vi "test_read-nmea-data2.vi"() -> ()   [LabVIEW 2019] (continued)
$GAGSV,2,1,08,02,08,297,,04,66,118,20,09,32,193,,11,71,358,,2*7E\n\t\n15:11:17.65\tF9P\t$GAGSV,2,2,08,12,40,102,24,19,26,045,24,25,09,249,,36,26,308,,2*7C\n\t\n15:11:17.67\tF9P\t$GBGSV,1,1,03,11,50,131,24,14,87,138,31,33,60,219,26,1*4F\n\t\n15:11:17.69\tF9P\t$GBGSV,1,1,03,11,50,131,31,14,87,138,23,33,60,219,,3*4E\n\t\n15:11:17.71\tF9P\t$GNGLL,3723.53985,N,12656.90241,E,061119.00,A,A*76\n\t\n15:11:17.73\tF9P\t\t\n15:11:17.75\tF9P\t\t\n15:11:17.77\tF9P\t\t\n15:11:17.79\tF9P\t\t\n15:11:17.81\tF9P\t\t\n15:11:17.83\tF9P\t\t\n15:11:17.85\tF9P\t\t\n15:11:17.87\tF9P\t\t\n15:11:17.89\tF9P\t\t\n15:11:17.91\tF9P\t\t\n15:11:17.93\tF9P\t\t\n15:11:17.95\tF9P\t\t\n15:11:17.97\tF9P\t\t\n15:11:17.99\tF9P\t\t\n15:11:18.01\tF9P\t\t\n15:11:18.03\tF9P\t\t\n15:11:18.05\tF9P\t\t\n15:11:18.07\tF9P\t\t\n15:11:18.09\tF9P\t\t\n15:11:18.11\tF9P\t\t\n15:11:18.13\tF9P\t\t\n15:11:18.15\tF9P\t\t\n15:11:18.17\tF9P\t\t\n15:11:18.19\tF9P\t\t\n15:11:18.21\tF9P\t\t\n15:11:18.23\tF9P\t\t\n15:11:18.25\tF9P\t$GNRMC,061120.00,A,3723.53889,N,12656.90285,E,2.155,137.19,250720,,,A,V*08\n\t\n15:11:18.27\tF9P\t$GNVTG,137.19,T,,M,2.155,N,3.990,K,A*2E\n\t\n15:11:18.29\tF9P\t$GNGGA,061120.00,3723.53889,N,12656.90285,E,1,12,0.68,42.0,M,18.5,M,,*7B\n\t\n15:11:18.31\tF9P\t$GNGSA,A,3,12,06,19,05,17,09,04,02,,,,,1.27,0.68,1.08,1*03\n\t\n15:11:18.33\tF9P\t$GNGSA,A,3,85,71,84,,,,,,,,,,1.27,0.68,1.08,2*06\n\t\n15:11:18.35\tF9P\t$GNGSA,A,3,36,19,11,04,09,12,,,,,,,1.27,0.68,1.08,3*03\n\t\n15:11:18.37\tF9P\t$GNGSA,A,3,14,11,33,,,,,,,,,,1.27,0.68,1.08,4*02\n\t\n15:11:18.39\tF9P\t$GPGSV,3,1,09,02,54,318,32,04,18,044,24,05,37,247,29,06,64,047,35,1*66\n\t\n15:11:18.41\tF9P\t$GPGSV,3,2,09,09,45,074,31,12,24,277,21,17,33,153,38,19,53,157,29,1*6D\n\t\n15:11:18.43\tF9P\t$GPGSV,3,3,09,25,12,307,16,1*5A\n\t\n15:11:18.45\tF9P\t$GPGSV,3,1,09,02,54,318,,04,18,044,21,05,37,247,,06,64,047,,6*68\n\t\n15:11:18.47\tF9P\t$GPGSV,3,2,09,09,45,074,23,12,24,277,,17,33,153,21,19,53,157,,6*69\n\t\n15:11:18.49\tF9P\t$GPGSV,3,3,09,25,12,307,,6*5A\n\t\n15:11:18.51\tF9P\t$GLGSV,2,1,08,69,12,031,,70,72,041,,71,51,205,20,72,03,209,,1*70\n\t\n15:11:18.53\tF9P\t$GLGSV,2,2,08,77,01,326,,84,20,122,10,85,70,065,23,86,36,330,,1*7B\n\t\n15:11:18.55\tF9P\t$GLGSV,2,1,08,69,12,031,,70,72,041,,71,51,205,15,72,03,209,,3*74\n\t\n15:11:18.57\tF9P\t$GLGSV,2,2,08,77,01,326,,84,20,122,18,85,70,065,20,86,36,330,,3*72\n\t\n15:11:18.59\tF9P\t$GAGSV,2,1,08,02,08,297,06,04,66,118,31,09,32,193,31,11,71,358,23,7*7E\n\t\n15:11:18.61\tF9P\t$GAGSV,2,2,08,12,40,102,22,19,26,045,22,25,09,249,,36,26,308,38,7*72\n\t\n15:11:18.63\tF9P\t$GAGSV,2,1,08,02,08,297,,04,66,118,20,09,32,193,,11,71,358,,2*7E\n\t\n15:11:18.65\tF9P\t$GAGSV,2,2,08,12,40,102,23,19,26,045,22,25,09,249,,36,26,308,,2*7D\n\t\n15:11:18.67\tF9P\t$GBGSV,1,1,03,11,50,132,24,14,87,138,26,33,60,219,25,1*49\n\t\n15:11:18.69\tF9P\t$GBGSV,1,1,03,11,50,132,24,14,87,138,22,33,60,219,,3*48\n\t\n15:11:18.71\tF9P\t$GNGLL,3723.53889,N,12656.90285,E,061120.00,A,A*79\n\t\n15:11:18.73\tF9P\t\t\n15:11:18.75\tF9P\t\t\n15:11:18.77\tF9P\t\t\n15:11:18.79\tF9P\t\t\n15:11:18.81\tF9P\t\t\n15:11:18.83\tF9P\t\t\n15:11:18.85\tF9P\t\t\n15:11:18.87\tF9P\t\t\n15:11:18.89\tF9P\t\t\n15:11:18.91\tF9P\t\t\n15:11:18.93\tF9P\t\t\n15:11:18.95\tF9P\t\t\n15:11:18.97\tF9P\t\t\n15:11:18.99\tF9P\t\t\n15:11:19.01\tF9P\t\t\n15:11:19.03\tF9P\t\t\n15:11:19.05\tF9P\t\t\n15:11:19.07\tF9P\t\t\n15:11:19.09\tF9P\t\t\n15:11:19.11\tF9P\t\t\n15:11:19.13\tF9P\t\t\n15:11:19.15\tF9P\t\t\n15:11:19.17\tF9P\t\t\n15:11:19.19\tF9P\t\t\n15:11:19.21\tF9P\t\t\n15:11:19.23\tF9P\t\t\n15:11:19.25\tF9P\t$GNRMC,061121.00,A,3723.53803,N,12656.90342,E,2.573,139.60,250720,,,A,V*01\n\t\n15:11:19.27\tF9P\t$GNVTG,139.60,T,,M,2.573,N,4.764,K,A*2C\n\t\n15:11:19.29\tF9P\t$GNGGA,061121.00,3723.53803,N,12656.90342,E,1,12,0.68,40.8,M,18.5,M,,*78\n\t\n15:11:19.31\tF9P\t$GNGSA,A,3,12,06,19,05,17,09,04,02,,,,,1.27,0.68,1.08,1*03\n\t\n15:11:19.33\tF9P\t$GNGSA,A,3,85,71,84,,,,,,,,,,1.27,0.68,1.08,2*06\n\t\n15:11:19.35\tF9P\t$GNGSA,A,3,36,19,11,04,09,12,,,,,,,1.27,0.68,1.08,3*03\n\t\n15:11:19.37\tF9P\t$GNGSA,A,3,14,11,33,,,,,,,,,,1.27,0.68,1.08,4*02\n\t\n15:11:19.39\tF9P\t$GPGSV,3,1,09,02,54,318,32,04,18,044,25,05,37,247,28,06,64,047,30,1*63\n\t\n15:11:19.41\tF9P\t$GPGSV,3,2,09,09,45,074,27,12,24,277,22,17,33,153,36,19,53,157,33,1*6C\n\t\n15:11:19.43\tF9P\t$GPGSV,3,3,09,25,12,307,16,1*5A\n\t\n15:11:19.45\tF9P\t$GPGSV,3,1,09,02,54,318,,04,18,044,21,05,37,247,,06,64,047,19,6*60\n\t\n15:11:19.47\tF9P\t$GPGSV,3,2,09,09,45,074,19,12,24,277,,17,33,153,22,19,53,157,,6*63\n\t\n15:11:19.49\tF9P\t$GPGSV,3,3,09,25,12,307,,6*5A\n\t\n15:11:19.51\tF9P\t$GLGSV,2,1,08,69,12,031,,70,72,041,,71,51,205,19,72,03,209,,1*7A\n\t\n15:11:19.53\tF9P\t$GLGSV,2,2,08,77,01,326,,84,20,122,10,85,70,065,23,86,36,330,,1*7B\n\t\n15:11:19.55\tF9P\t$GLGSV,2,1,08,69,12,031,,70,72,041,,71,51,205,16,72,03,209,,3*77\n\t\n15:11:19.57\tF9P\t$GLGSV,2,2,08,77,01,326,,84,20,122,18,85,70,065,19,86,36,330,,3*78\n\t\n15:11:19.59\tF9P\t$GAGSV,2,1,08,02,08,297,10,04,66,118,30,09,32,193,30,11,71,358,28,7*72\n\t\n15:11:19.61\tF9P\t$GAGSV,2,2,08,12,40,102,21,19,26,045,22,25,09,249,,36,26,308,23,7*7B\n\t\n15:11:19.63\tF9P\t$GAGSV,2,1,08,02,08,297,,04,66,118,20,09,32,193,,11,71,358,,2*7E\n\t\n15:11:19.65\tF9P\t$GAGSV,2,2,08,12,40,102,23,19,26,045,18,25,09,249,,36,26,308,,2*74\n\t\n15:11:19.67\tF9P\t$GBGSV,1,1,03,11,50,132,24,14,87,127,23,33,60,219,23,1*44\n\t\n15:11:19.69\tF9P\t$GBGSV,1,1,03,11,50,132,25,14,87,127,22,33,60,219,,3*47\n\t\n15:11:19.71\tF9P\t$GNGLL,3723.53803,N,12656.90342,E,061121.00,A,A*70\n\t\n15:11:19.73\tF9P\t\t\n15:11:19.75\tF9P\t\t\n15:11:19.77\tF9P\t\t\n15:11:19.79\tF9P\t\t\n15:11:19.81\tF9P\t\t\n15:11:19.83\tF9P\t\t\n15:11:19.85\tF9P\t\t\n15:11:19.87\tF9P\t\t\n15:11:19.89\tF9P\t\t\n15:11:19.91\tF9P\t\t\n15:11:19.93\tF9P\t\t\n15:11:19.95\tF9P\t\t\n15:11:19.97\tF9P\t\t\n15:11:19.99\tF9P\t\t\n15:11:20.01\tF9P\t\t\n15:11:20.03\tF9P\t\t\n15:11:20.05\tF9P\t\t\n15:11:20.07\tF9P\t\t\n15:11:20.09\tF9P\t\t\n15:11:20.11\tF9P\t\t\n15:11:20.13\tF9P\t\t\n15:11:20.15\tF9P\t\t\n15:11:20.17\tF9P\t\t\n15:11:20.19\tF9P\t\t\n15:11:20.21\tF9P\t\t\n15:11:20.23\tF9P\t\t\n15:11:20.25\tF9P\t$GNRMC,061122.00,A,3723.53728,N,12656.90355,E,1.979,141.75,250720,,,A,V*0C\n\t\n15:11:20.27\tF9P\t$GNVTG,141.75,T,,M,1.979,N,3.666,K,A*26\n\t\n15:11:20.29\tF9P\t$GNGGA,061122.00,3723.53728,N,12656.90355,E,1,12,0.67,41.8,M,18.5,M,,*75\n\t\n15:11:20.31\tF9P\t$GNGSA,A,3,12,06,19,05,17,09,04,02,,,,,1.28,0.67,1.09,1*02\n\t\n15:11:20.33\tF9P\t$GNGSA,A,3,85,71,84,,,,,,,,,,1.28,0.67,1.09,2*07\n\t\n15:11:20.35\tF9P\t$GNGSA,A,3,36,19,11,04,09,12,,,,,,,1.28,0.67,1.09,3*02\n\t\n15:11:20.37\tF9P\t$GNGSA,A,3,14,11,33,,,,,,,,,,1.28,0.67,1.09,4*03\n\t\n15:11:20.39\tF9P\t$GPGSV,3,1,09,02,54,318,32,04,18,044,23,05,37,247,28,06,64,047,29,1*6D\n\t\n15:11:20.41\tF9P\t$GPGSV,3,2,09,09,45,074,31,12,24,277,21,17,33,153,34,19,53,157,33,1*6A\n\t\n15:11:20.43\tF9P\t$GPGSV,3,3,09,25,12,307,15,1*59\n\t\n15:11:20.45\tF9P\t$GPGSV,3,1,09,02,54,318,,04,18,044,20,05,37,247,21,06,64,047,20,6*68\n\t\n15:11:20.47\tF9P\t$GPGSV,3,2,09,09,45,074,20,12,24,277,,17,33,153,29,19,53,157,,6*62\n\t\n15:11:20.49\tF9P\t$GPGSV,3,3,09,25,12,307,,6*5A\n\t\n15:11:20.51\tF9P\t$GLGSV,2,1,08,69,12,031,,70,72,041,,71,51,205,21,72,03,209,,1*71\n\t\n15:11:20.53\tF9P\t$GLGSV,2,2,08,77,01,326,,84,20,122,12,85,70,065,29,86,36,330,,1*73\n\t\n15:11:20.55\tF9P\t$GLGSV,2,1,08,69,12,031,,70,72,041,,71,51,205,17,72,03,209,,3*76\n\t\n15:11:20.57\tF9P\t$GLGSV,2,2,08,77,01,326,,84,20,122,18,85,70,065,19,86,36,330,,3*78\n\t\n15:11:20.59\tF9P\t$GAGSV,2,1,08,02,08,297,11,04,66,118,30,09,32,193,30,11,71,358,14,7*7C\n\t\n15:11:20.61\tF9P\t$GAGSV,2,2,08,12,40,102,23,19,26,045,21,25,09,249,,36,26,308,30,7*78\n\t\n15:11:20.63\tF9P\t$GAGSV,2,1,08,02,08,297,,04,66,118,30,09,32,193,,11,71,358,,2*7F\n\t\n15:11:20.65\tF9P\t$GAGSV,2,2,08,12,40,102,21,19,26,045,15,25,09,249,,36,26,308,,2*7B\n\t\n15:11:20.67\tF9P\t$GBGSV,1,1,03,11,50,132,24,14,87,127,22,33,60,219,22,1*44\n\t\n15:11:20.69\tF9P\t$GBGSV,1,1,03,11,50,132,,14,87,127,23,33,60,219,,3*41\n\t\n15:11:20.71\tF9P\t$GNGLL,3723.53728,N,12656.90355,E,061122.00,A,A*73\n\t\n15:11:20.73\tF9P\t\t\n15:11:20.75\tF9P\t\t\n15:11:20.77\tF9P\t\t\n15:11:20.79\tF9P\t\t\n15:11:20.81\tF9P\t\t\n15:11:20.83\tF9P\t\t\n15:11:20.85\tF9P\t\t\n15:11:20.87\tF9P\t\t\n15:11:20.89\tF9P\t\t\n15:11:20.91\tF9P\t\t\n15:11:20.93\tF9P\t\t\n15:11:20.95\tF9P\t\t\n15:11:20.97\tF9P\t\t\n15:11:20.99\tF9P\t\t\n15:11:21.01\tF9P\t\t\n15:11:21.03\tF9P\t\t\n15:11:21.05\tF9P\t\t\n15:11:21.07\tF9P\t\t\n15:11:21.09\tF9P\t\t\n15:11:21.11\tF9P\t\t\n15:11:21.13\tF9P\t\t\n15:11:21.15\tF9P\t\t\n15:11:21.17\tF9P\t\t\n15:11:21.19\tF9P\t\t\n15:11:21.21\tF9P\t\t\n15:11:21.23\tF9P\t\t\n15:11:21.25\tF9P\t$GNRMC,061123.00,A,3723.53633,N,12656.90395,E,2.590,146.65,250720,,,A,V*04\n\t\n15:11:21.27\tF9P\t$GNVTG,146.65,T,,M,2.590,N,4.796,K,A*21\n\t\n15:11:21.29\tF9P\t$GNGGA,061123.00,3723.53633,N,12656.90395,E,1,12,0.64,39.9,M,18.5,M,,*7E\n\t\n15:11:21.31\tF9P\t$GNGSA,A,3,12,06,19,05,17,09,04,02,,,,,1.18,0.64,0.99,1*0A\n\t\n15:11:21.33\tF9P\t$GNGSA,A,3,85,71,84,,,,,,,,,,1.18,0.64,0.99,2*0F\n\t\n15:11:21.35\tF9P\t$GNGSA,A,3,36,19,11,04,09,12,,,,,,,1.18,0.64,0.99,3*0A\n\t\n15:11:21.37\tF9P\t$GNGSA,A,3,14,11,33,,,,,,,,,,1.18,0.64,0.99,4*0B\n\t\n15:11:21.39\tF9P\t$GPGSV,3,1,09,02,54,318,35,04,18,044,23,05,37,247,33,06,64,047,30,1*68\n\t\n15:11:21.41\tF9P\t$GPGSV,3,2,09,09,45,074,27,12,24,277,21,17,33,153,37,19,53,157,27,1*6B\n\t\n15:11:21.43\tF9P\t$GPGSV,3,3,09,25,12,307,15,1*59\n\t\n15:11:21.45\tF9P\t$GPGSV,3,1,09,02,54,318,,04,18,044,18,05,37,247,20,06,64,047,20,6*62\n\t\n15:11:21.47\tF9P\t$GPGSV,3,2,09,09,45,074,22,12,24,277,,17,33,153,21,19,53,157,,6*68\n\t\n15:11:21.49\tF9P\t$GPGSV,3,3,09,25,12,307,,6*5A\n\t\n15:11:21.51\tF9P\t$GLGSV,2,1,08,69,12,031,,70,72,041,,71,51,205,21,72,03,209,,1*71\n\t\n15:11:21.53\tF9P\t$GLGSV,2,2,08,77,01,326,,84,20,122,12,85,70,065,24,86,36,330,,1*7E\n\t\n15:11:21.55\tF9P\t$GLGSV,2,1,08,69,12,031,,70,72,041,,71,51,205,18,72,03,209,,3*79\n\t\n15:11:21.57\tF9P\t$GLGSV,2,2,08,77,01,326,,84,20,122,20,85,70,065,19,86,36,330,,3*73\n\t\n15:11:21.59\tF9P\t$GAGSV,2,1,08,02,08,297,09,04,66,118,33,09,32,193,31,11,71,358,25,7*75\n\t\n15:11:21.61\tF9P\t$GAGSV,2,2,08,12,40,102,24,19,26,045,20,25,09,249,,36,26,308,33,7*7D\n\t\n15:11:21.63\tF9P\t$GAGSV,2,1,08,02,08,297,,04,66,118,,09,32,193,,11,71,358,,2*7C\n\t\n15:11:21.65\tF9P\t$GAGSV,2,2,08,12,40,102,22,19,26,045,14,25,09,249,,36,26,308,,2*79\n\t\n15:11:21.67\tF9P\t$GBGSV,1,1,03,11,50,132,25,14,87,127,23,33,60,219,21,1*47\n\t\n15:11:21.69\tF9P\t$GBGSV,1,1,03,11,50,132,25,14,87,127,,33,60,219,,3*47\n\t\n15:11:21.71\tF9P\t$GNGLL,3723.53633,N,12656.90395,E,061123.00,A,A*75\n\t\n15:11:21.73\tF9P\t\t\n15:11:21.75\tF9P\t\t\n15:11:21.77\tF9P\t\t\n15:11:21.79\tF9P\t\t\n15:11:21.81\tF9P\t\t\n15:11:21.83\tF9P\t\t\n15:11:21.85\tF9P\t\t\n15:11:21.87\tF9P\t\t\n15:11:21.89\tF9P\t\t\n15:11:21.91\tF9P\t\t\n15:11:21.93\tF9P\t\t\n15:11:21.95\tF9P\t\t\n15:11:21.97\tF9P\t\t\n15:11:21.99\tF9P\t\t\n15:11:22.01\tF9P\t\t\n15:11:22.03\tF9P\t\t\n15:11:22.05\tF9P\t\t\n15:11:22.07\tF9P\t\t\n15:11:22.09\tF9P\t\t\n15:11:22.11\tF9P\t\t\n15:11:22.13\tF9P\t\t\n15:11:22.15\tF9P\t\t\n15:11:22.17\tF9P\t\t\n15:11:22.19\tF9P\t\t\n15:11:22.21\tF9P\t\t\n15:11:22.23\tF9P\t\t\n15:11:22.25\tF9P\t$GNRMC,061124.00,A,3723.53563,N,12656.90459,E,2.521,142.29,250720,,,A,V*04\n\t\n15:11:22.27\tF9P\t$GNVTG,142.29,T,,M,2.521,N,4.669,K,A*26\n\t\n15:11:22.29\tF9P\t$GNGGA,061124.00,3723.53563,N,12656.90459,E,1,12,0.64,38.0,M,18.5,M,,*70\n\t\n15:11:22.31\tF9P\t$GNGSA,A,3,12,06,19,05,17,09,04,02,,,,,1.18,0.64,0.99,1*0A\n\t\n15:11:22.33\tF9P\t$GNGSA,A,3,85,71,84,,,,,,,,,,1.18,0.64,0.99,2*0F\n\t\n15:11:22.35\tF9P\t$GNGSA,A,3,36,19,11,04,09,12,,,,,,,1.18,0.64,0.99,3*0A\n\t\n15:11:22.37\tF9P\t$GNGSA,A,3,14,11,33,,,,,,,,,,1.18,0.64,0.99,4*0B\n\t\n15:11:22.39\tF9P\t$GPGSV,3,1,09,02,54,318,35,04,18,044,22,05,37,247,32,06,64,047,34,1*6C\n\t\n15:11:22.41\tF9P\t$GPGSV,3,2,09,09,45,074,31,12,24,277,21,17,33,153,36,19,53,157,31,1*6A\n\t\n15:11:22.43\tF9P\t$GPGSV,3,3,09,25,12,307,14,1*58\n\t\n15:11:22.45\tF9P\t$GPGSV,3,1,09,02,54,318,,04,18,044,16,05,37,247,17,06,64,047,20,6*68\n\t\n15:11:22.47\tF9P\t$GPGSV,3,2,09,09,45,074,22,12,24,277,,17,33,153,23,19,53,157,,6*6A\n\t\n15:11:22.49\tF9P\t$GPGSV,3,3,09,25,12,307,,6*5A\n\t\n15:11:22.51\tF9P\t$GLGSV,2,1,08,69,12,031,,70,72,041,,71,51,205,21,72,03,209,,1*71\n\t\n15:11:22.53\tF9P\t$GLGSV,2,2,08,77,01,326,,84,20,122,10,85,70,065,22,86,36,330,,1*7A\n\t\n15:11:22.55\tF9P\t$GLGSV,2,1,08,69,12,031,,70,72,041,,71,51,205,21,72,03,209,,3*73\n\t\n15:11:22.57\tF9P\t$GLGSV,2,2,08,77,01,326,,84,20,122,19,85,70,065,20,86,36,330,,3*73\n\t\n15:11:22.59\tF9P\t$GAGSV,2,1,08,02,08,297,11,04,66,118,28,09,32,193,24,11,71,358,24,7*73\n\t\n15:11:22.61\tF9P\t$GAGSV,2,2,08,12,40,102,23,19,26,045,17,25,09,249,,36,26,308,34,7*79\n\t\n15:11:22.63\tF9P\t$GAGSV,2,1,08,02,08,297,,04,66,118,,09,32,193,,11,71,358,,2*7C\n\t\n15:11:22.65\tF9P\t$GAGSV,2,2,08,12,40,102,21,19,26,045,10,25,09,249,,36,26,308,,2*7E\n\t\n15:11:22.67\tF9P\t$GBGSV,1,1,03,11,50,132,25,14,87,127,24,33,60,219,22,1*43\n\t\n15:11:22.69\tF9P\t$GBGSV,1,1,03,11,50,132,30,14,87,127,23,33,60,219,,3*42\n\t\n15:11:22.71\tF9P\t$GNGLL,3723.53563,N,12656.90459,E,061124.00,A,A*73\n\t\n15:11:22.73\tF9P\t\t\n15:11:22.75\tF9P\t\t\n15:11:22.77\tF9P\t\t\n15:11:22.79\tF9P\t\t\n15:11:22.81\tF9P\t\t\n15:11:22.83\tF9P\t\t\n15:11:22.85\tF9P\t\t\n15:11:22.87\tF9P\t\t\n15:11:22.89\tF9P\t\t\n15:11:22.91\tF9P\t\t\n15:11:22.93\tF9P\t\t\n15:11:22.95\tF9P\t\t\n15:11:22.97\tF9P\t\t\n15:11:22.99\tF9P\t\t\n15:11:23.01\tF9P\t\t\n15:11:23.03\tF9P\t\t\n15:11:23.05\tF9P\t\t\n15:11:23.07\tF9P\t\t\n15:11:23.09\tF9P\t\t\n15:11:23.11\tF9P\t\t\n15:11:23.13\tF9P\t\t\n15:11:23.15\tF9P\t\t\n15:11:23.17\tF9P\t\t\n15:11:23.19\tF9P\t\t\n15:11:23.21\tF9P\t\t\n15:11:23.23\tF9P\t\t\n15:11:23.25\tF9P\t$GNRMC,061125.00,A,3723.53464,N,12656.90520,E,2.575,142.58,250720,,,A,V*0B\n\t\n15:11:23.27\tF9P\t$GNVTG,142.58,T,,M,2.575,N,4.768,K,A*21\n\t\n15:11:23.29\tF9P\t$GNGGA,061125.00,3723.53464,N,12656.90520,E,1,12,0.71,36.2,M,18.5,M,,*70\n\t\n15:11:23.31\tF9P\t$GNGSA,A,3,12,06,19,05,17,09,04,02,,,,,1.35,0.71,1.15,1*04\n\t\n15:11:23.33\tF9P\t$GNGSA,A,3,85,71,84,,,,,,,,,,1.35,0.71,1.15,2*01\n\t\n15:11:23.35\tF9P\t$GNGSA,A,3,36,19,11,04,09,12,,,,,,,1.35,0.71,1.15,3*04\n\t\n15:11:23.37\tF9P\t$GNGSA,A,3,14,11,33,,,,,,,,,,1.35,0.71,1.15,4*05\n\t\n15:11:23.39\tF9P\t$GPGSV,3,1,09,02,54,318,30,04,18,044,21,05,37,247,31,06,64,047,29,1*65\n\t\n15:11:23.41\tF9P\t$GPGSV,3,2,09,09,45,074,26,12,24,277,23,17,33,153,38,19,53,157,27,1*67\n\t\n15:11:23.43\tF9P\t$GPGSV,3,3,09,25,12,307,14,1*58\n\t\n15:11:23.45\tF9P\t$GPGSV,3,1,09,02,54,318,,04,18,044,13,05,37,247,19,06,64,047,20,6*63\n\t\n15:11:23.47\tF9P\t$GPGSV,3,2,09,09,45,074,21,12,24,277,,17,33,153,22,19,53,157,,6*68\n\t\n15:11:23.49\tF9P\t$GPGSV,3,3,09,25,12,307,,6*5A\n\t\n15:11:23.51\tF9P\t$GLGSV,2,1,08,69,12,031,,70,72,041,,71,51,205,23,72,03,209,,1*73\n\t\n15:11:23.53\tF9P\t$GLGSV,2,2,08,77,01,326,,84,20,122,10,85,70,065,23,86,36,330,,1*7B\n\t\n15:11:23.55\tF9P\t$GLGSV,2,1,08,69,12,031,,70,72,041,,71,51,205,22,72,03,209,,3*70\n\t\n15:11:23.57\tF9P\t$GLGSV,2,2,08,77,01,326,,84,20,122,18,85,70,065,18,86,36,330,,3*79\n\t\n15:11:23.59\tF9P\t$GAGSV,2,1,08,02,08,297,10,04,66,118,26,09,32,193,30,11,71,358,22,7*7F\n\t\n15:11:23.61\tF9P\t$GAGSV,2,2,08,12,40,102,23,19,26,045,16,25,09,249,,36,26,308,26,7*7B\n\t\n15:11:23.63\tF9P\t$GAGSV,2,1,08,02,08,297,,04,66,118,,09,32,193,,11,71,358,,2*7C\n\t\n15:11:23.65\tF9P\t$GAGSV,2,2,08,12,40,102,28,19,26,045,08,25,09,249,,36,26,308,,2*7E\n\t\n15:11:23.67\tF9P\t$GBGSV,1,1,03,11,50,132,24,14,87,127,23,33,60,219,22,1*45\n\t\n15:11:23.69\tF9P\t$GBGSV,1,1,03,11,50,132,,14,87,127,22,33,60,219,,3*40\n\t\n15:11:23.71\tF9P\t$GNGLL,3723.53464,N,12656.90520,E,061125.00,A,A*7B\n\t\n15:11:23.73\tF9P\t\t\n15:11:23.75\tF9P\t\t\n15:11:23.77\tF9P\t\t\n15:11:23.79\tF9P\t\t\n15:11:23.81\tF9P\t\t\n15:11:23.83\tF9P\t\t\n15:11:23.85\tF9P\t\t\n15:11:23.87\tF9P\t\t\n15:11:23.89\tF9P\t\t\n15:11:23.91\tF9P\t\t\n15:11:23.93\tF9P\t\t\n15:11:23.95\tF9P\t\t\n15:11:23.97\tF9P\t\t\n15:11:23.99\tF9P\t\t\n15:11:24.01\tF9P\t\t\n15:11:24.03\tF9P\t\t\n15:11:24.05\tF9P\t\t\n15:11:24.07\tF9P\t\t\n15:11:24.09\tF9P\t\t\n15:11:24.11\tF9P\t\t\n15:11:24.13\tF9P\t\t\n15:11:24.15\tF9P\t\t\n15:11:24.17\tF9P\t\t\n15:11:24.19\tF9P\t\t\n15:11:24.21\tF9P\t\t\n15:11:24.23\tF9P\t\t\n15:11:24.25\tF9P\t$GNRMC,061126.00,A,3723.53410,N,12656.90564,E,1.876,133.23,250720,,,A,V*0C\n\t\n15:11:24.27\tF9P\t$GNVTG,133.23,T,,M,1.876,N,3.475,K,A*2E\n\t\n15:11:24.29\tF9P\t$GNGGA,061126.00,3723.53410,N,12656.90564,E,1,12,0.68,36.0,M,18.5,M,,*7A\n\t\n15:11:24.31\tF9P\t$GNGSA,A,3,12,06,19,05,17,09,04,02,,,,,1.26,0.68,1.05,1*0F\n\t\n15:11:24.33\tF9P\t$GNGSA,A,3,85,71,84,,,,,,,,,,1.26,0.68,1.05,2*0A\n\t\n15:11:24.35\tF9P\t$GNGSA,A,3,36,19,11,04,09,12,,,,,,,1.26,0.68,1.05,3*0F\n\t\n15:11:24.37\tF9P\t$GNGSA,A,3,14,11,33,,,,,,,,,,1.26,0.68,1.05,4*0E\n\t\n15:11:24.39\tF9P\t$GPGSV,3,1,09,02,54,318,34,04,18,044,20,05,37,247,26,06,64,047,29,1*66\n\t\n15:11:24.41\tF9P\t$GPGSV,3,2,09,09,45,074,32,12,24,277,22,17,33,153,34,19,53,157,27,1*6F\n\t\n15:11:24.43\tF9P\t$GPGSV,3,3,09,25,12,307,14,1*58\n\t\n15:11:24.45\tF9P\t$GPGSV,3,1,09,02,54,318,,04,18,044,11,05,37,247,20,06,64,047,21,6*6A\n\t\n15:11:24.47\tF9P\t$GPGSV,3,2,09,09,45,074,23,12,24,277,,17,33,153,23,19,53,157,,6*6B\n\t\n15:11:24.49\tF9P\t$GPGSV,3,3,09,25,12,307,,6*5A\n\t\n15:11:24.51\tF9P\t$GLGSV,2,1,08,69,12,031,,70,72,041,,71,51,205,24,72,03,209,,1*74\n\t\n15:11:24.53\tF9P\t$GLGSV,2,2,08,77,01,326,,84,20,122,09,85,70,065,22,86,36,330,,1*72\n\t\n15:11:24.55\tF9P\t$GLGSV,2,1,08,69,12,031,,70,72,041,,71,51,205,23,72,03,209,,3*71\n\t\n15:11:24.57\tF9P\t$GLGSV,2,2,08,77,01,326,,84,20,122,17,85,70,065,18,86,36,330,,3*76\n\t\n15:11:24.59\tF9P\t$GAGSV,2,1,08,02,08,297,10,04,66,118,27,09,32,193,32,11,71,358,24,7*7A\n\t\n15:11:24.61\tF9P\t$GAGSV,2,2,08,12,40,102,23,19,26,045,16,25,09,249,,36,26,308,27,7*7A\n\t\n15:11:24.63\tF9P\t$GAGSV,2,1,08,02,08,297,,04,66,118,,09,32,193,,11,71,358,,2*7C\n\t\n15:11:24.65\tF9P\t$GAGSV,2,2,08,12,40,102,,19,26,045,09,25,09,249,,36,26,308,,2*75\n\t\n15:11:24.67\tF9P\t$GBGSV,1,1,03,11,50,132,26,14,87,127,23,33,60,219,23,1*46\n\t\n15:11:24.69\tF9P\t$GBGSV,1,1,03,11,50,132,26,14,87,127,21,33,60,219,,3*47\n\t\n15:11:24.71\tF9P\t$GNGLL,3723.53410,N,12656.90564,E,061126.00,A,A*7B\n\t\n15:11:24.73\tF9P\t\t\n15:11:24.75\tF9P\t\t\n15:11:24.77\tF9P\t\t\n15:11:24.79\tF9P\t\t\n15:11:24.81\tF9P\t\t\n15:11:24.83\tF9P\t\t\n15:11:24.85\tF9P\t\t\n15:11:24.87\tF9P\t\t\n15:11:24.89\tF9P\t\t\n15:11:24.91\tF9P\t\t\n15:11:24.93\tF9P\t\t\n15:11:24.95\tF9P\t\t\n15:11:24.97\tF9P\t\t\n15:11:24.99\tF9P\t\t\n15:11:25.01\tF9P\t\t\n15:11:25.03\tF9P\t\t\n15:11:25.05\tF9P\t\t\n15:11:25.07\tF9P\t\t\n15:11:25.09\tF9P\t\t\n15:11:25.11\tF9P\t\t\n15:11:25.13\tF9P\t\t\n15:11:25.15\tF9P\t\t\n15:11:25.17\tF9P\t\t\n15:11:25.19\tF9P\t\t\n15:11:25.21\tF9P\t\t\n15:11:25.23\tF9P\t\t\n15:11:25.25\tF9P\t$GNRMC,061127.00,A,3723.53368,N,12656.90596,E,1.809,132.45,250720,,,A,V*01\n\t\n15:11:25.27\tF9P\t$GNVTG,132.45,T,,M,1.809,N,3.351,K,A*26\n\t\n15:11:25.29\tF9P\t$GNGGA,061127.00,3723.53368,N,12656.90596,E,1,12,0.72,35.5,M,18.5,M,,*73\n\t\n15:11:25.31\tF9P\t$GNGSA,A,3,12,06,19,05,17,09,04,02,,,,,1.36,0.72,1.15,1*04\n\t\n15:11:25.33\tF9P\t$GNGSA,A,3,85,71,84,,,,,,,,,,1.36,0.72,1.15,2*01\n\t\n15:11:25.35\tF9P\t$GNGSA,A,3,36,19,11,04,09,12,,,,,,,1.36,0.72,1.15,3*04\n\t\n15:11:25.37\tF9P\t$GNGSA,A,3,14,11,33,,,,,,,,,,1.36,0.72,1.15,4*05\n\t\n15:11:25.39\tF9P\t$GPGSV,3,1,09,02,54,318,32,04,18,044,19,05,37,247,29,06,64,047,29,1*65\n\t\n15:11:25.41\tF9P\t$GPGSV,3,2,09,09,45,074,28,12,24,277,21,17,33,153,35,19,53,157,25,1*64\n\t\n15:11:25.43\tF9P\t$GPGSV,3,3,09,25,12,307,16,1*5A\n\t\n15:11:25.45\tF9P\t$GPGSV,3,1,09,02,54,318,,04,18,044,,05,37,247,20,06,64,047,21,6*6A\n\t\n15:11:25.47\tF9P\t$GPGSV,3,2,09,09,45,074,31,12,24,277,,17,33,153,24,19,53,157,,6*6F\n\t\n15:11:25.49\tF9P\t$GPGSV,3,3,09,25,12,307,,6*5A\n\t\n15:11:25.51\tF9P\t$GLGSV,2,1,08,69,12,031,,70,72,041,,71,51,
